vi "Camera_List.vi"(10 "设备":u16(ring) items=["设备1_22592_3034", "设备2_22592_3034"], 11 "error in":errorcluster) -> (4 "获取设备列表返回值":i32, 6 "DevCfgGet":cluster{"pid":u32, "vid":u32, "ser_num":u64}[](array[cluster]), 8 "设备列表":i32[](array[numeric]), 15 "error out":errorcluster)   [LabVIEW 2016]
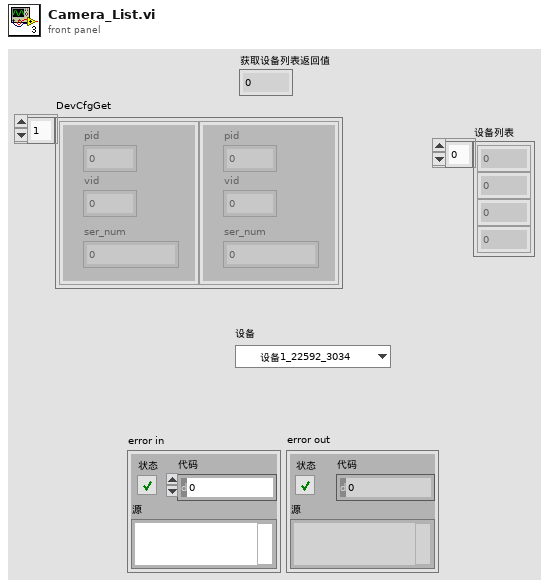
[diagram p1: front panel]
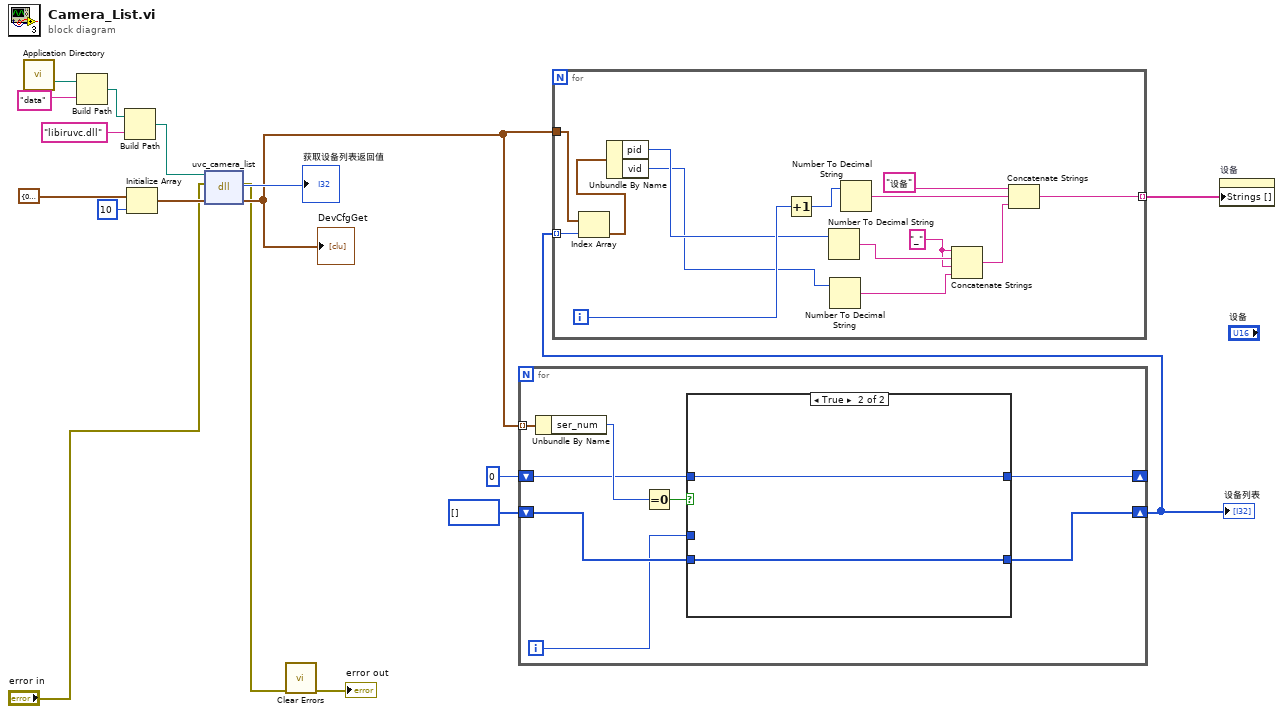
[diagram p0: block diagram]
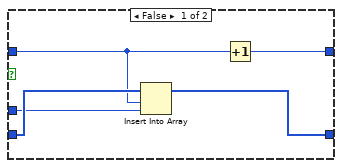
[diagram p2: hidden frame]
diagram:
  n1 = call <vilib>:"Application Directory.vi"() -> ("Application Directory"=w14:path)
  n2 = Build Path(base path=w14, name or relative path="data") -> (appended path=w17:path)
  n3 = Build Path(base path=w17, name or relative path="libiruvc.dll") -> (appended path=w12:path)
  n4 = Initialize Array(cluster{"pid":u32, "vid":u32, "ser_num":u64} {"pid"=0, "vid"=0, "ser_num"=0} ("DevCfg"), 10 ("dimension size")) -> (w10:cluster{"pid":u32, "vid":u32, "ser_num":u64}[])
  n5 = dll-call lib="D:/libiruvc_0.3.3/windows/x64/dll/libiruvc.dll" fn="uvc_camera_list"(path in=w12, error in="error in", "devs_cfg[]"=w10) -> (error out=w3:errorcluster, "return type"=→"获取设备列表返回值":i32, "devs_cfg[]"=w5:cluster{"pid":u32, "vid":u32, "ser_num":u64}[])  [unwired: 1 in, 1 out]
  "DevCfgGet" <- w5
  n6 = call <vilib>:"Clear Errors.vi"("error in (no error)"=w3) -> ("error out"=→"error out":errorcluster)  [unwired: 5 in, 1 out]
  n7 = for {
    tunnel: w5 -> [w25] mode=indexing
    shift-right: [w19] -> w8
    shift-left: i32[] [] -> [w22]
    shift-right: [w20] -> _
    shift-left: 0 -> [w21]
    i -> [w18]
    n8 = Unbundle By Name(w25) -> ("ser_num"=w23:u64)
    n9 = Equal To 0?(x=w23) -> (x = 0?=w24:bool)
    n10 = case shown="True" w24 {
      tunnel: w22 -> [w30 w31]
      tunnel: w21 -> [w28 w32]
      tunnel: [w27 w32] -> w20
      tunnel: [w26 w31] -> w19
      tunnel: w18 -> [w29 _]
      frame False {
        n11 = Insert Into Array(array=w30, index=w28, new element=w29) -> (w26:i32[])
        n12 = Increment(x=w28) -> (x+1=w27:i32)
      }
      frame True {
      }
    }
  }
  "设备列表" <- w8
  n13 = for {
    tunnel: w8 -> [w43] mode=indexing
    tunnel: w5 -> [w42]
    tunnel: [w33] -> w7 mode=indexing
    i -> [w46]
    w36 = "_" ("string")
    n14 = Index Array(array=w42, index=w43) -> (element=w41:cluster{"pid":u32, "vid":u32, "ser_num":u64})
    n15 = Unbundle By Name(w41) -> ("pid"=w45:u32, "vid"=w44:u32)
    n16 = Increment(x=w46) -> (x+1=w38:i32)
    n17 = Number To Decimal String(number=w45) -> (decimal integer string=w37:string)  [unwired: 1 in]
    n18 = Number To Decimal String(number=w44) -> (decimal integer string=w35:string)  [unwired: 1 in]
    n19 = Number To Decimal String(number=w38) -> (decimal integer string=w40:string)  [unwired: 1 in]
    n20 = Concatenate Strings(w36, w37, w36, w35) -> (w34:string)
    n21 = Concatenate Strings("设备", w40, w34) -> (w33:string)
  }
  n22 = property on="设备" class="Ring (strict)"("Strings []"=w7) -> ()  [unwired: 2 in, 2 out]
